vi "Get Normal Mode Data.vi"(8 "error in":errorcluster) -> (0 "error out":errorcluster, 3 "Potentiometer":fxp<+,18,3> format="%.16g")   [LabVIEW 2024, in "FPGA Interface.lvlib"]
uses:
  FPGA Interface.lvlib
  <vilib>/rvi/interface/nirviReadWriteControl/nirviReadWriteControl.xnode
  FPGA Bitfiles/ecu-9030_FPGATarget_FPGAMain_pDLqQGhG1UY.lvbitx
  Type Definitions/ECU FPGA Reference.ctl
  FPGA Reference - Get.vi
  NiFpgaLv.dll
  <vilib>/Utility/error.llb/Error Cluster From Error Code.vi
  <vilib>/rvi/errors/niLvFpgaAdjustHostInterfaceError.vi
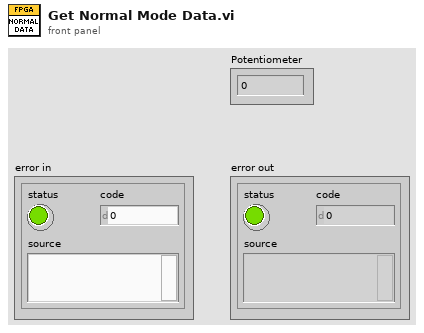
[diagram p1: front panel]
types:
  T1 = typedef "ECU FPGA Reference.ctl" = refnum<k20>
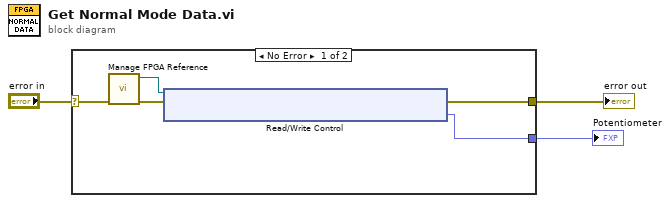
[diagram p0: block diagram]
diagram:
  n1 = case shown="No Error" "error in" {
    selector: "error in" -> [w5 w9]
    tunnel: [w8 w9] -> w3
    tunnel: [w4 _] -> w1
    frame No Error {
      n2 = call-poly "Manage FPGA Reference.vi"("error in"=w5) -> ("error out"=w6:errorcluster, "FPGA Reference Out"=w7:T1)  [unwired: 9 in]
      n3 = xnode "Read/Write Control"("FPGA VI Reference In"=w7, "error in"=w6) -> ("error out"=w8:errorcluster, "Potentiometer"=w4:fxp<+,18,3>)  [unwired: 1 out]
    }
    frame Error {
    }
  }
  "error out" <- w3
  "Potentiometer" <- w1
